vi "Introspection Core.vi"(8 "error in (no error)":errorcluster, 11 "CS++DIM-Server in":refnum<class "CS++DIM-Server.lvclass">) -> (0 "error out":errorcluster, 2 "CS++Messages":refnum<class "Message.lvclass">[](array[class]), 3 "CS++DIM-Server out":refnum<class "CS++DIM-Server.lvclass">)   [LabVIEW 2014, in "CS++DIM-Server.lvlib" / "CS++DIM-Server.lvclass"]
doc: "This vi delivers a list with all messages this actor reacts to. \n\nNote that all inherited classes have to overwrite it."
uses:
  CS++DIM-Server.lvclass
  <vilib>/ActorFramework/Message/Message.lvclass
  CSPP_Core/Actors/CS++BaseActor/CS++BaseActor.lvclass
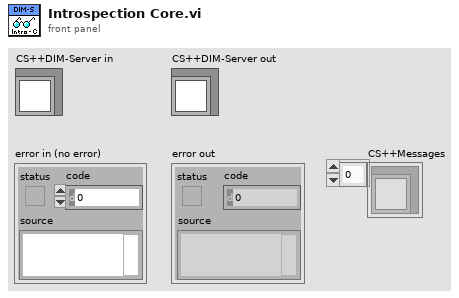
[diagram p1: front panel]
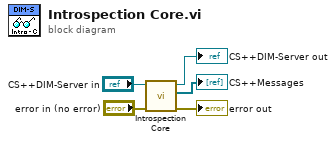
[diagram p0: block diagram]
diagram:
  n1 = call-parent "Introspection Core.vi"("error in (no error)"="error in (no error)", "CS++BaseActor in"="CS++DIM-Server in") -> ("error out"=→"error out":errorcluster, "CS++Messages"=→"CS++Messages":refnum<class "Message.lvclass">[], "CS++BaseActor out"=→"CS++DIM-Server out":refnum<class "CS++DIM-Server.lvclass">)  [unwired: 7 in]
